vi "ZP Conditions and Checking.vi"(0 "Input Points":dbl[](array[numeric]) format="%.2f", 1 "Zeros-Poles-Gains":T1(array[cluster]) {"Poles" format="%.2f"; "Zeros" format="%.2f"; "gain" format="%.2f"}) -> (2 "previous samples":dbl[](array[numeric]) format="%.2f", 3 "additive constants":dbl[](array[numeric]) format="%.2f", 4 "internal states":cluster{dbl[]}[](array[cluster]) {"?" format="%.2f"}, 5 "numerators":cluster{"Numerator new":dbl[]}[](array[cluster]) {"Numerator new" format="%.2f"}, 6 "denominators":cluster{"Denominator new":dbl[]}[](array[cluster]) {"Denominator new" format="%.2f"}, 7 "gains":dbl[](array[numeric]) format="%.2f")   [LabVIEW 2020, in "NI_AdvCtrl_continuous linear.lvlib"]
doc: "LabVIEW no longer supports this VI. You can obtain similar functionality by installing the LabVIEW Simulation Module."
uses:
  <vilib>/addons/control/advanced/NI_AdvCtrl_continuous linear.lvlib
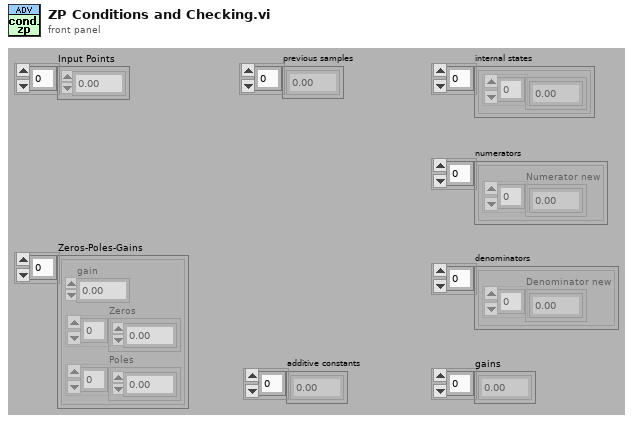
[diagram p1: front panel]
types:
  T1 = cluster{"gain":dbl, "Zeros":cdb[], "Poles":cdb[]}[]
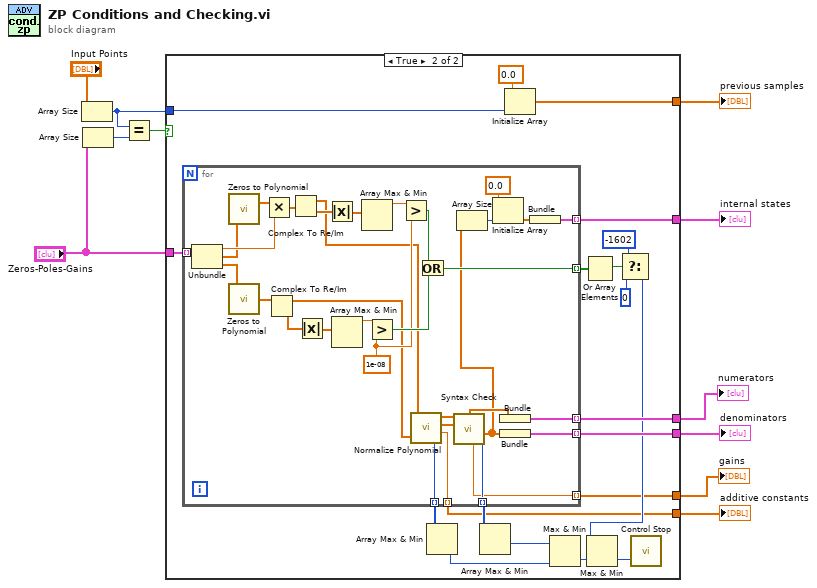
[diagram p0: block diagram]
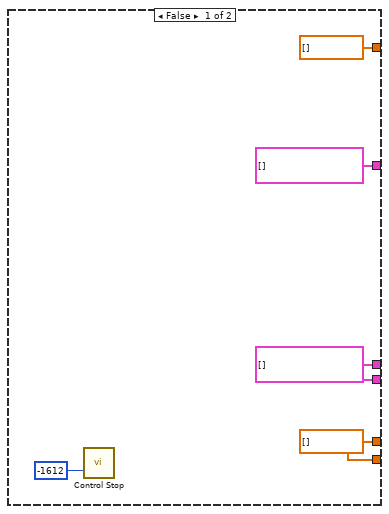
[diagram p2: hidden frame]
diagram:
  n1 = Array Size(array="Input Points") -> (size(s)=w9:i32)
  n2 = Array Size(array="Zeros-Poles-Gains") -> (size(s)=w11:i32)
  n3 = Equal?(x=w9, y=w11) -> (x = y?=w1:bool)
  n4 = case shown="True" w1 {
    tunnel: "Zeros-Poles-Gains" -> [_ w36]
    tunnel: w9 -> [_ w35]
    tunnel: [cluster{dbl[]}[] [] w34] -> w8
    tunnel: [w14 w33] -> w7
    tunnel: [w14 w32] -> w6
    tunnel: [dbl[] [] w31] -> w5
    tunnel: [w15 w18] -> w3
    tunnel: [w15 w17] -> w2
    frame False {
      w14 = cluster{"Numerator new":dbl[]}[] []
      w15 = dbl[] []
      n5 = call <vilib>:"Control Stop.vi"("error"=-1612 ("f")) -> ()  [unwired: 2 out]
    }
    frame True {
      n6 = for {
        tunnel: [w69] -> w21 mode=indexing
        tunnel: [w68] -> w17 mode=indexing
        tunnel: [w65] -> w20 mode=indexing
        tunnel: [w64] -> w18 mode=indexing
        tunnel: [w49] -> w19 mode=indexing
        tunnel: w36 -> [w48] mode=indexing
        tunnel: [w39] -> w32 mode=indexing
        tunnel: [w38] -> w33 mode=indexing
        tunnel: [w37] -> w34 mode=indexing
        w58 = 1e-08
        n7 = Unbundle(w48) -> ("gain"=w47:dbl, "Zeros"=w46:cdb[], "Poles"=w45:cdb[])
        n8 = call <vilib>:"Zeros to Polynomial.vi"("Zeros"=w46) -> ("Polynomial"=w54:cdb[])
        n9 = call <vilib>:"Zeros to Polynomial.vi"("Zeros"=w45) -> ("Polynomial"=w53:cdb[])
        n10 = Multiply(x=w54, y=w47) -> (x*y=w52:cdb[])
        n11 = Complex To Re/Im(x + iy=w53) -> (x=w50:dbl[], y=w56:dbl[])
        n12 = Complex To Re/Im(x + iy=w52) -> (x=w51:dbl[], y=w62:dbl[])
        n13 = Absolute Value(x=w56) -> (abs(x)=w55:dbl[])
        n14 = Absolute Value(x=w62) -> (abs(x)=w61:dbl[])
        n15 = Array Max & Min(array=w55) -> (max value=w57:dbl)  [unwired: 3 out]
        n16 = Array Max & Min(array=w61) -> (max value=w63:dbl)  [unwired: 3 out]
        n17 = Greater?(x=w57, y=w58) -> (0:w59:bool)
        n18 = Greater?(x=w63, y=w58) -> (0:w60:bool)
        n19 = call <vilib>:"Normalize Polynomial.vi"("Numerator"=w51, "Denominator"=w50) -> ("Numerator new"=w66:dbl[], "Denominator new"=w67:dbl[], "additive constant"=w68:dbl, "error"=w69:i32)
        n20 = Or(x=w60, y=w59) -> (x .or. y?=w49:bool)
        n21 = call <vilib>:"Syntax Check.vi"("Denominator"=w67, "Numerator"=w66) -> ("error"=w65:i32, "gain"=w64:dbl, "Denominator new"=w40:dbl[], "Numerator new"=w44:dbl[])  [unwired: 1 out]
        n22 = Array Size(array=w40) -> (size(s)=w42:i32)
        n23 = Initialize Array(0.0, w42) -> (w41:dbl[])
        n24 = Bundle("Numerator new"=w44) -> (w39:cluster{"Numerator new":dbl[]})  [unwired: 1 in]
        n25 = Bundle("Denominator new"=w40) -> (w38:cluster{"Denominator new":dbl[]})  [unwired: 1 in]
        n26 = Bundle(w41) -> (w37:cluster{dbl[]})  [unwired: 1 in]
      }
      n27 = Array Max & Min(array=w21) -> (min value=w23:i32)  [unwired: 3 out]
      n28 = Array Max & Min(array=w20) -> (min value=w22:i32)  [unwired: 3 out]
      n29 = Initialize Array(0.0 ("Element Data"), w35) -> (w31:dbl[])
      n30 = Max & Min(x=w22, y=w23) -> (min(x,y)=w24:i32)  [unwired: 1 out]
      n31 = Or Array Elements(Boolean array=w19) -> (logical OR=w26:bool)
      n32 = Select(t=-1602, s=w26, f=0) -> (s? t:f=w27:i32)
      n33 = Max & Min(x=w27, y=w24) -> (min(x,y)=w25:i32)  [unwired: 1 out]
      n34 = call <vilib>:"Control Stop.vi"("error"=w25) -> ()  [unwired: 2 out]
    }
  }
  "internal states" <- w8
  "denominators" <- w7
  "numerators" <- w6
  "previous samples" <- w5
  "gains" <- w3
  "additive constants" <- w2
